vi "runAnalyer.vi"(8 "error in (no error)":errorcluster, 10 "closeEvent":refnum<user-event>, 11 "ImageAnalyser in":refnum<class "ImageAnalyser.lvclass">) -> (0 "error out":errorcluster, 3 "ImageAnalyser out":refnum<class "ImageAnalyser.lvclass">)   [LabVIEW 2011, in "Tools.lvlib" / "Imaging.lvlib" / "ImageAnalyser.lvclass"]
uses:
  ImageAnalyser.lvclass
  FluorescenceLiveAnalyser/FluorescenceLiveAnalyser.lvclass
panel:
  in  "stop":bool
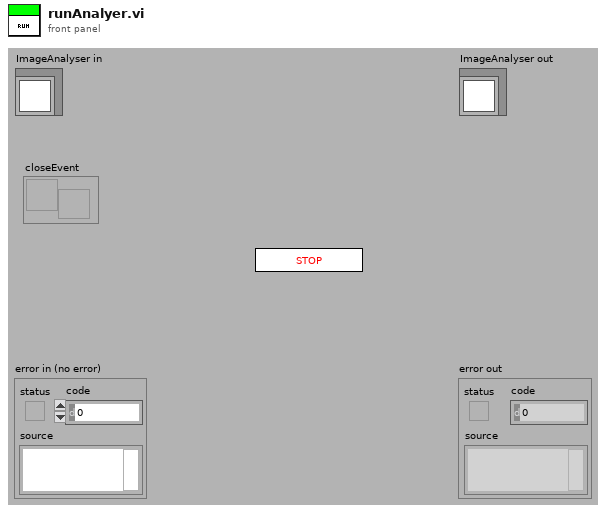
[diagram p1: front panel]
types:
  T1 = cluster{"ImageName":string, "ImageArray":sgl[][]}
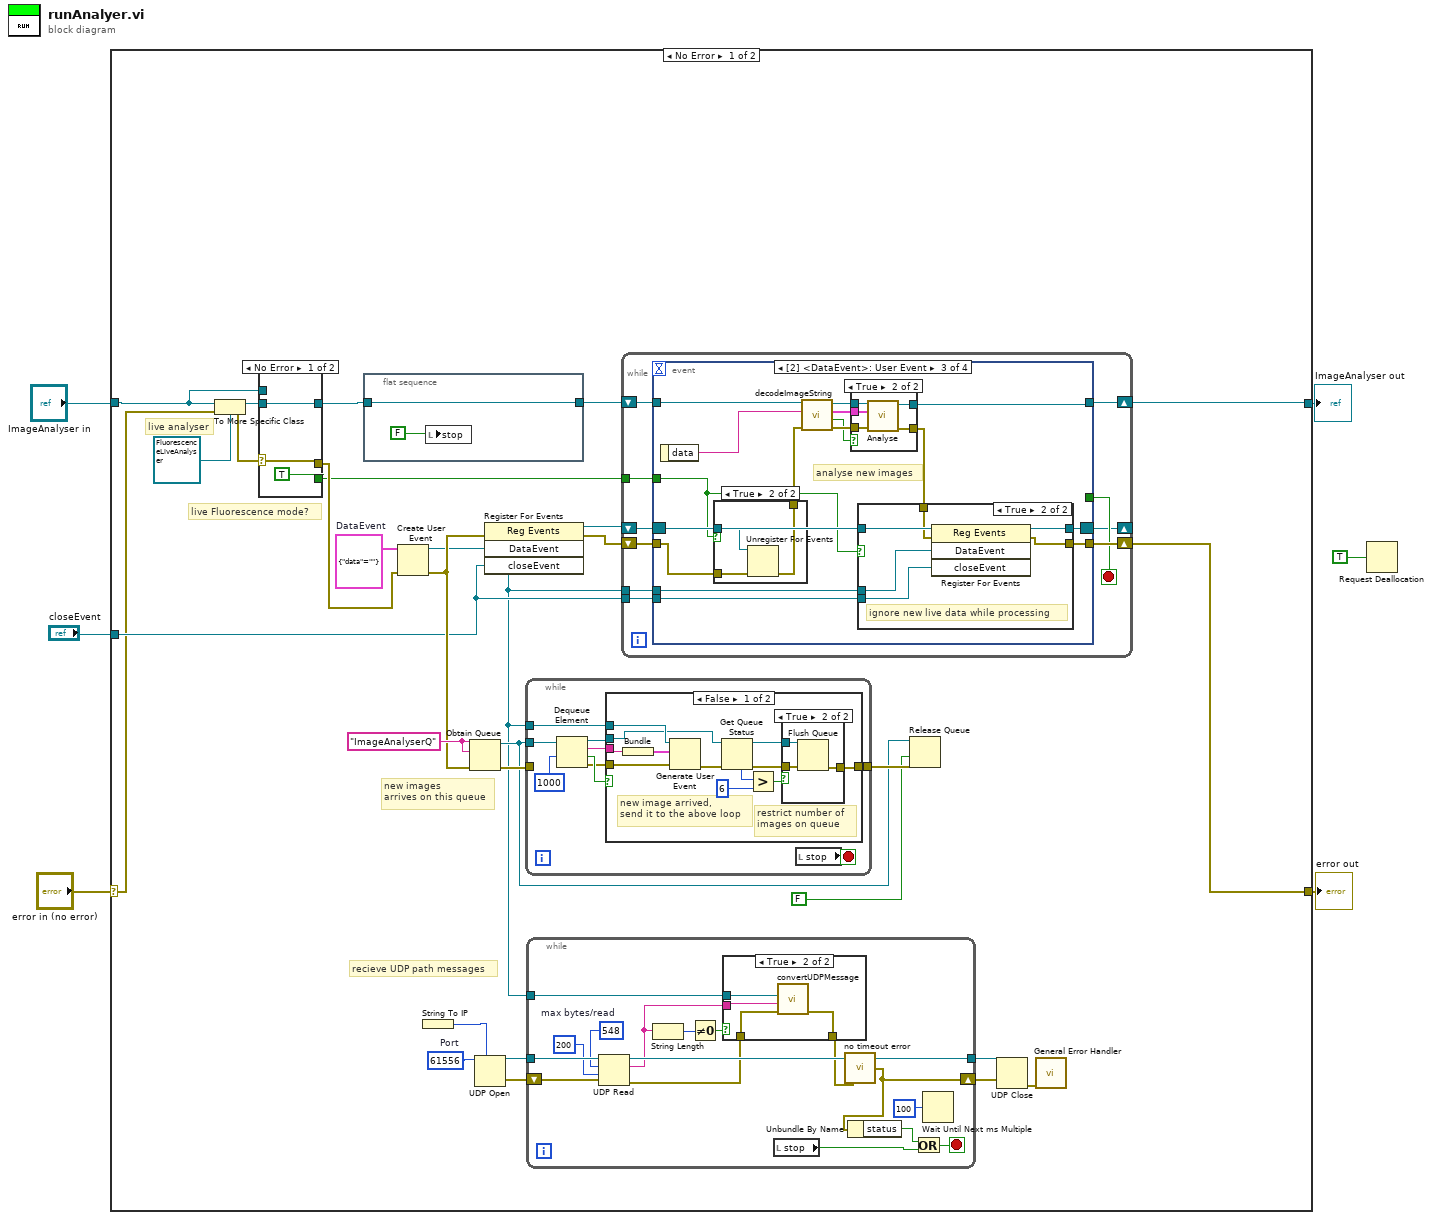
[diagram p0: block diagram]
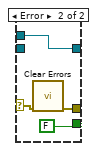
[diagram p2: hidden frame]
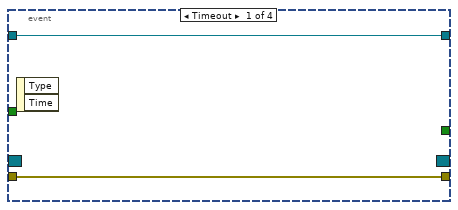
[diagram p4: hidden frame]
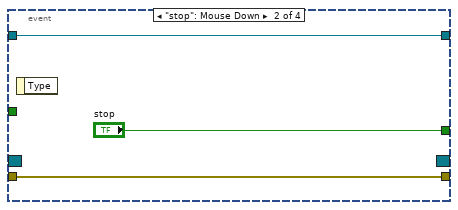
[diagram p5: hidden frame]
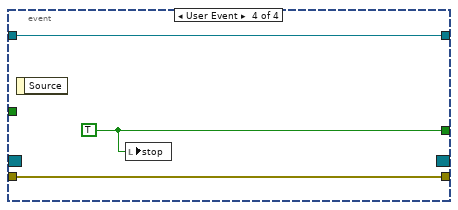
[diagram p9: hidden frame]
diagram:
  n1 = case shown="No Error" "error in (no error)" {
    selector: "error in (no error)" -> [w12 w146]
    tunnel: [w23 w146] -> w5
    tunnel: [w31 w145] -> w3
    tunnel: "ImageAnalyser in" -> [w8 w145]
    tunnel: "closeEvent" -> [w24 _]
    frame No Error {
      w22 = u16 61556  # Port
      w29 = cluster{"data":string} {"data"=""}  # DataEvent
      w30 = "ImageAnalyserQ"
      # "live analyser"
      # "live Fluorescence mode?"
      # "recieve UDP path messages"
      # "new images\narrives on this queue"
      n2 = To More Specific Class(target class=refnum<class "FluorescenceLiveAnalyser.lvclass"> refnum ("Tools.lvlib:Imaging.lvlib:FluorescenceLiveAnalyser.lvclass"), reference=w8, error in=w12) -> (specific class reference=w9:refnum<class "FluorescenceLiveAnalyser.lvclass">, error out=w14:errorcluster)
      n3 = case shown="No Error" w14 {
        selector: w14 -> [w38 w42]
        tunnel: [w38 w41] -> w11
        tunnel: [TRUE FALSE] -> w10
        tunnel: w9 -> [w36 _]
        tunnel: w8 -> [_ w39]
        tunnel: [w36 w39] -> w7
        frame No Error {
        }
        frame Error {
          n4 = call <vilib>:"Clear Errors.vi"("error in (no error)"=w42) -> ("error out"=w41:errorcluster)  [unwired: 6 in]
        }
      }
      n5 = flat-sequence {
        tunnel: [w65] -> w25
        tunnel: w7 -> [w65]
        frame #0 {
          n6 = local write "stop"(FALSE) -> ()
        }
      }
      n7 = Create User Event(user event datatype=w29, error in=w11) -> (user event=w16:refnum<user-event>, error out=w27:errorcluster)
      n8 = String To IP() -> (0:w15:u32)  [unwired: 1 in]
      n9 = Obtain Queue(name (unnamed)=w30, element data type=w30, error in (no error)=w27) -> (queue out=w33:refnum<queue>, error out=w35:errorcluster)  [unwired: 2 in, 1 out]
      n10 = UDP Open(7:w15, 11:w22) -> (port=w20:refnum<k16>, 0:w21:errorcluster)  [unwired: 3 in, 1 out]
      n11 = register-events(error in=w27, w16, w24) -> (reference out=w28:refnum<event-registration>, error out=w26:errorcluster)  [unwired: 1 in]
      n12 = while {
        tunnel: w33 -> [w127]
        tunnel: w35 -> [_]
        tunnel: [w124] -> w34
        tunnel: w16 -> [w121]
        stop <- w123 stop-if-true
        n13 = Dequeue Element(queue=w127, timeout in ms (-1)=1000) -> (queue out=w119:refnum<queue>, element=w122:string, timed out?=w126:bool, error out=w125:errorcluster)  [unwired: 1 in]
        n14 = case shown="False" w126 {
          tunnel: w125 -> [w139 w144]
          tunnel: [w128 w144] -> w124
          tunnel: w122 -> [w138 _]
          tunnel: w121 -> [w137 _]
          tunnel: w119 -> [w134 _]
          frame False {
            # "restrict number of \nimages on queue"
            # "new image arrived, \nsend it to the above loop"
            n15 = Bundle(w138) -> (w136:cluster{string})  [unwired: 1 in]
            n16 = Generate User Event(user event=w137, event data cluster=w136, error in=w139) -> (error out=w135:errorcluster)  [unwired: 1 out]
            n17 = Get Queue Status(queue=w134, error in (no error)=w135) -> (queue out=w129:refnum<queue>, error out=w130:errorcluster, # elements in queue=w133:i32)  [unwired: 1 in, 5 out]
            n18 = Greater?(x=w133, y=6) -> (0:w131:bool)
            n19 = case shown="True" w131 {
              tunnel: w130 -> [w140 w143]
              tunnel: w129 -> [_ w141]
              tunnel: [w140 w142] -> w128
              frame False {
              }
              frame True {
                n20 = Flush Queue(queue=w141, error in (no error)=w143) -> (error out=w142:errorcluster)  [unwired: 2 out]
              }
            }
          }
          frame True {
            # "timeout"
          }
        }
        n21 = local read "stop"() -> (w123:bool)
      }
      n22 = while {
        tunnel: [w56] -> w19
        tunnel: w20 -> [w57]
        shift-left: w21 -> [w58]
        shift-right: [w52] -> w18
        tunnel: w16 -> [w43]
        stop <- w54 stop-if-true
        w51 = 548  # max bytes/read
        n23 = UDP Read(connection ID=w57, max size (548)=w51, timeout ms (25000)=200, 8:w58) -> (data out=w49:string, error out=w46:errorcluster, 3:w56:refnum<k16>)  [unwired: 2 out]
        n24 = String Length(string=w49) -> (length=w48:i32)
        n25 = Not Equal To 0?(x=w48) -> (x != 0?=w47:bool)
        n26 = case shown="True" w47 {
          tunnel: w49 -> [_ w60]
          tunnel: w46 -> [w59 w62]
          tunnel: [w59 w61] -> w45
          tunnel: w43 -> [_ w63]
          frame False {
          }
          frame True {
            n27 = call "convertUDPMessage.vi"("error in (no error)"=w62, "message"=w60, "user event out"=w63) -> ("error out"=w61:errorcluster)  [unwired: 8 in]
          }
        }
        n28 = local read "stop"() -> (w44:bool)
        n29 = call "no timeout error.vi"("error in (no error)"=w45) -> ("error out"=w52:errorcluster)
        n30 = Unbundle By Name(w52) -> ("status"=w53:bool)
        n31 = Or(x=w53, y=w44) -> (x .or. y?=w54:bool)
        n32 = Wait Until Next ms Multiple(millisecond multiple=u32 100) -> ()  [unwired: 1 out]
      }
      n33 = while {
        shift-right: [w75] -> w31
        shift-left: w25 -> [w74]
        shift-right: [w71] -> w23
        shift-left: w26 -> [w72]
        tunnel: w16 -> [w69]
        tunnel: w24 -> [w68]
        shift-right: [w67] -> _
        shift-left: w28 -> [w73]
        tunnel: w10 -> [w66]
        stop <- w70 stop-if-true
        n34 = event shown="[2] <DataEvent>: User Event" {
          selector: w73 -> [_ _ w87 _]
          dyn-events: [_ _ w83 _] -> w67
          timeout: _ -> [_ _ _ _]
          tunnel: [w77 w78 w93 w118] -> w75
          tunnel: w74 -> [w77 w78 w96 w118]
          tunnel: w72 -> [w76 w80 w89 w117]
          tunnel: [w76 w80 w84 w117] -> w71
          tunnel: [_ "stop" _ w116] -> w70
          tunnel: w69 -> [_ _ w86 _]
          tunnel: w68 -> [_ _ w85 _]
          tunnel: w66 -> [_ _ w81 _]
          event Timeout {
            n35 = event-data() -> ()  [unwired: 1 in, 2 out]
          }
          event "stop": Mouse Down {
            n36 = event-data() -> ()  [unwired: 1 in, 1 out]
          }
          event User Event {
            # "analyse new images"
            n37 = event-data() -> ("data"=w95:string)  [unwired: 1 in]
            n38 = case shown="True" w81 {
              tunnel: w89 -> [w105 w108]
              tunnel: [w105 w107] -> w88
              tunnel: w87 -> [_ w106]
              frame False {
              }
              frame True {
                n39 = Unregister For Events(event registration refnum=w106, error in=w108) -> (error out=w107:errorcluster)
              }
            }
            n40 = call "decodeImageString.vi"("error in (no error)"=w88, "encodedImage"=w95, "ImageAnalyser in"=w96) -> ("error out"=w92:errorcluster, "isImage?"=w91:bool, "ImageData"=w90:T1, "ImageAnalyser out"=w94:refnum<class "ImageAnalyser.lvclass">)  [unwired: 5 in]
            n41 = case shown="True" w91 {
              tunnel: w94 -> [w110 w115]
              tunnel: [w110 w114] -> w93
              tunnel: w92 -> [w109 w113]
              tunnel: [w109 w112] -> w82
              tunnel: w90 -> [_ w111]
              frame False {
              }
              frame True {
                n42 = call-dynamic "Analyse.vi"("error in (no error)"=w113, "ImageData"=w111, "ImageAnalyser in"=w115) -> ("error out"=w112:errorcluster, "ImageAnalyser out"=w114:refnum<class "ImageAnalyser.lvclass">)  [unwired: 7 in]
              }
            }
            n43 = case shown="True" w81 {
              tunnel: w87 -> [w98 w104]
              tunnel: w86 -> [_ w103]
              tunnel: w85 -> [_ w102]
              tunnel: [w97 w101] -> w84
              tunnel: [w98 w100] -> w83
              tunnel: w82 -> [w97 w99]
              frame False {
              }
              frame True {
                # "ignore new live data while processing"
                n44 = register-events(reference=w104, error in=w99, w103, w102) -> (reference out=w100:refnum<event-registration>, error out=w101:errorcluster)
              }
            }
          }
          event User Event {
            w116 = TRUE
            n45 = event-data() -> ()  [unwired: 1 in, 1 out]
            n46 = local write "stop"(w116) -> ()
          }
        }
      }
      n47 = Release Queue(queue=w33, force destroy? (F)=FALSE, error in (no error)=w34) -> ()  [unwired: 3 out]
      n48 = UDP Close(connection ID=w19, 8:w18) -> (error out=w17:errorcluster)  [unwired: 1 out]
      n49 = call <vilib>:"General Error Handler.vi"("error in (no error)"=w17) -> ()  [unwired: 10 in, 5 out]
    }
    frame Error {
    }
  }
  "error out" <- w5
  "ImageAnalyser out" <- w3
  n50 = Request Deallocation(TRUE ("flag")) -> ()
